vi "Many Stepper Mover Com.vi"() -> (0 "Command text":string[][](array[string]))   [LabVIEW 2019]
uses:
  Stepper Mover.ctl
panel:
  in  "Top or Bottom":T1(radio)
  in  "Initial Value":dbl
  in  "Final Value":dbl
  in  "Number of Interval":dbl
  in  "Generate":bool
  in  "cancel":bool
  in  "next":bool
  in  "Stepper Mover":T2={"extra wait"=0, "Stepper Value"=1.0, "Top or Bottom"=enum."Move to Top Position (deg)"} {"extra wait" min=0; "Stepper Value" format="%#.7e"}
  in  "wait after sweep (sec)":i32
  out "loop array":dbl[][](array[numeric])
  in  "Array":dbl[][](array[numeric]) format="%#_4e"
  # "Stepper Mover (Multiple Input Generator)"
  # "(Stepper Mover.vi needs to be open.)"
  # "generates multiple stepper mover values for the sequence, see belolw.  If you like it click \"Good, use this!\". You can also modify the values directly from the following array."
  # "Value"
  # "Stepper Mover"
  # "(Stepper Mover.vi needs to be open before using this program)"
  # "Value"
  # "seconds"
  # "AND wait extra"
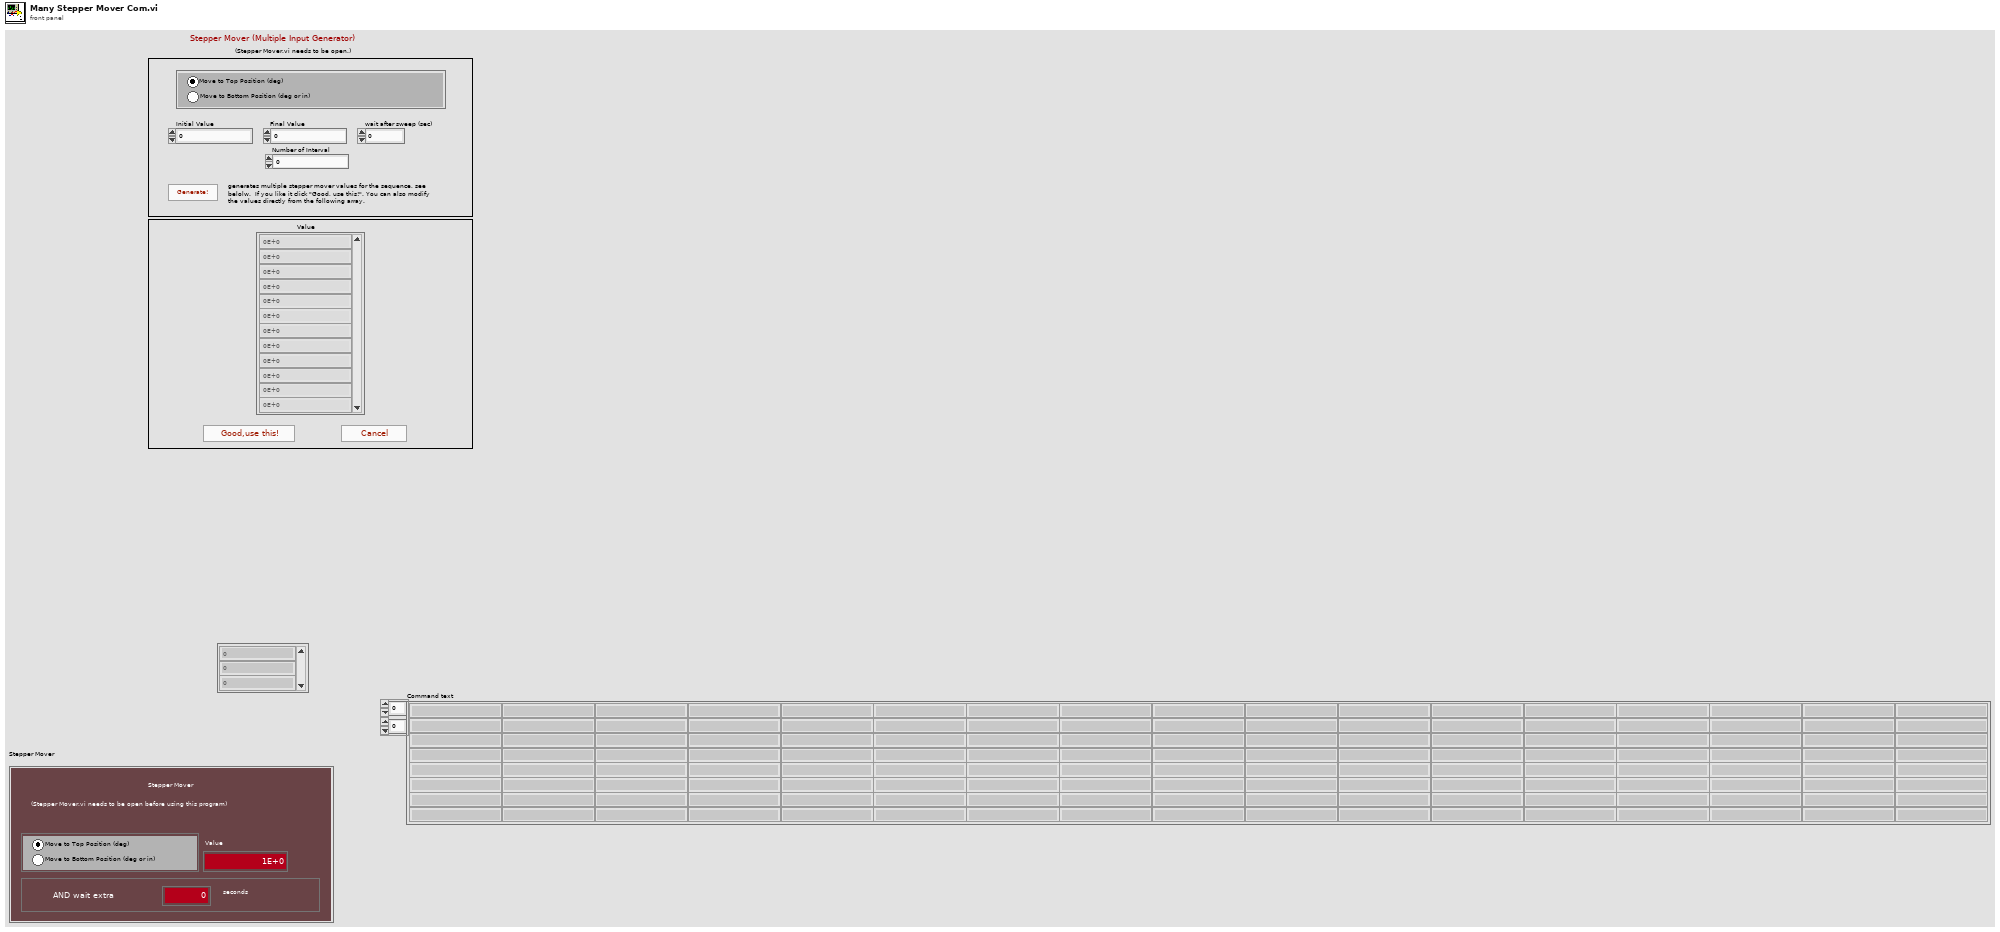
[diagram p1: front panel]
types:
  T1 = enum32{"Move to Top Position (deg)", "Move to Bottom Position (deg or in)"}
  T2 = typedef "Stepper Mover.ctl" = cluster{"extra wait":i32, "Stepper Value":dbl, "Top or Bottom":enum32{"Move to Top Position (deg)", "Move to Bottom Position (deg or in)"}}
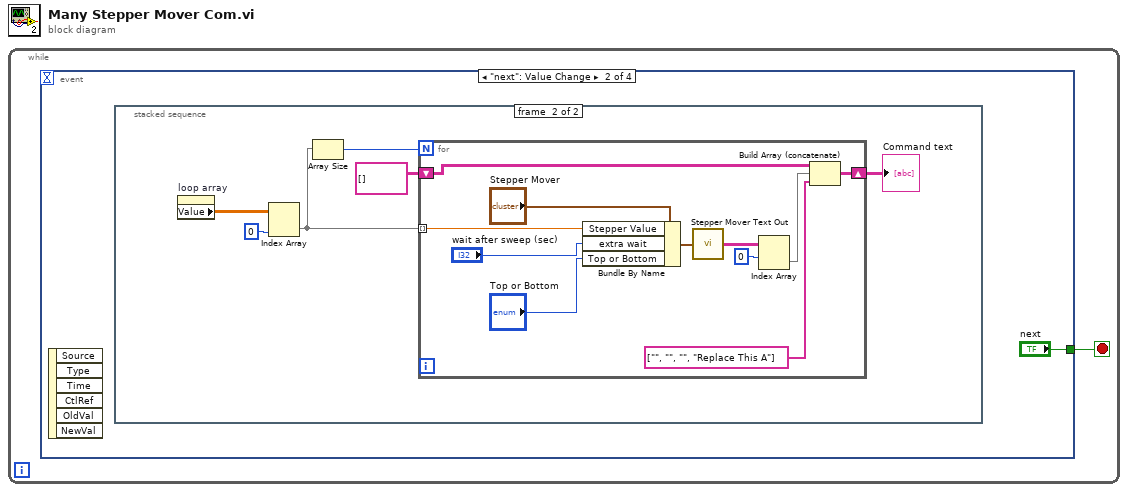
[diagram p0: block diagram]
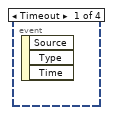
[diagram p2: hidden frame]
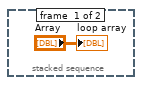
[diagram p3: hidden frame]
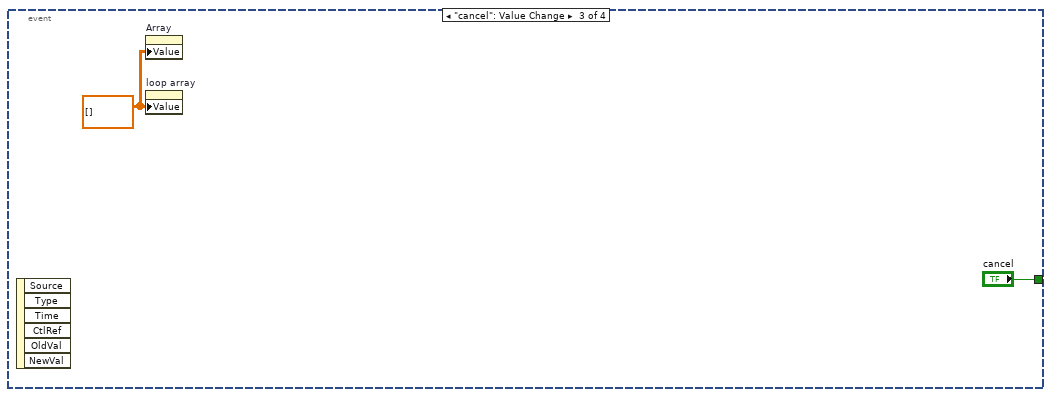
[diagram p4: hidden frame]
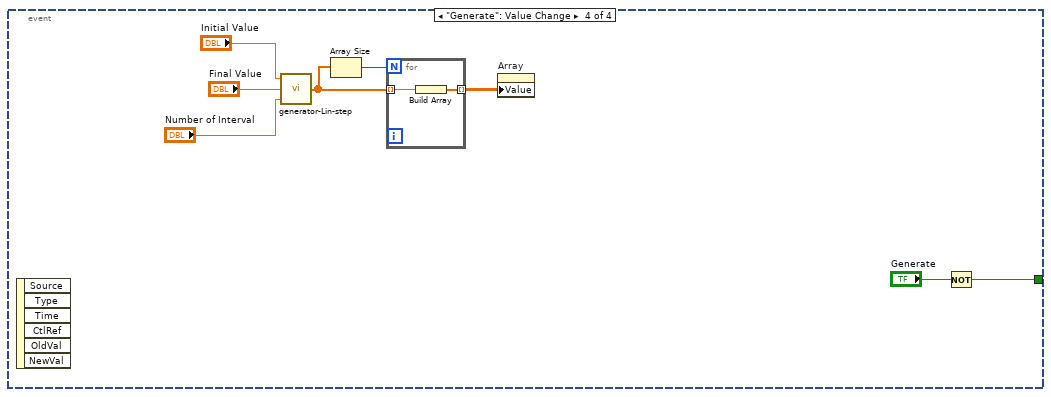
[diagram p5: hidden frame]
diagram:
  n1 = while {
    stop <- w1 stop-if-true
    n2 = event shown="[1] \"next\": Value Change" {
      selector: _ -> [_ _ _ _]
      dyn-events: _ -> [_ _ _ _]
      timeout: _ -> [_ _ _ _]
      tunnel: [_ "next" "cancel" w25] -> w1
      event Timeout {
        n3 = event-data() -> ()  [unwired: 1 in, 3 out]
      }
      event "next": Value Change {
        n4 = event-data() -> ()  [unwired: 1 in, 6 out]
        n5 = stacked-sequence {
          frame #0 {
            "loop array" <- "Array"
          }
          frame #1 {
            n6 = property on="loop array" class="Arr (strict)"() -> ("Value"=w8:dbl[][])  [unwired: 2 in, 2 out]
            n7 = Index Array(array=w8, index (col)=0 ("disabled index (col)")) -> (element=w7:dbl[])  [unwired: 1 in]
            n8 = Array Size(array=w7) -> (size(s)=w6:i32)
            n9 = for {
              N: w6 -> [_]
              tunnel: w7 -> [w11] mode=indexing
              shift-right: [w13] -> w5
              shift-left: string[][] [] -> [w12]
              n10 = Bundle By Name(cluster="Stepper Mover", "Stepper Value"=w11, "extra wait"="wait after sweep (sec)", "Top or Bottom"="Top or Bottom") -> (w19:T2)
              n11 = call "Stepper Mover Text Out.vi"("Stepper Mover"=w19) -> ("Command text"=w17:string[][])
              n12 = Index Array(array=w17, index (row)=0) -> (element=w15:string[])  [unwired: 1 in]
              n13 = Build Array (concatenate)(w12, w15, string[] ["", "", "", "Replace This A"]) -> (w13:string[][])
            }
            "Command text" <- w5
          }
        }
      }
      event "cancel": Value Change {
        w21 = dbl[][] [] ("Array")
        n14 = event-data() -> ()  [unwired: 1 in, 6 out]
        n15 = property on="Array" class="Arr (strict)"("Value"=w21) -> ()  [unwired: 2 in, 2 out]
        n16 = property on="loop array" class="Arr (strict)"("Value"=w21) -> ()  [unwired: 2 in, 2 out]
      }
      event "Generate": Value Change {
        n17 = event-data() -> ()  [unwired: 1 in, 6 out]
        n18 = call "generator-Lin-step.vi"("step"="Number of Interval", "end"="Final Value", "start"="Initial Value") -> ("Array"=w24:dbl[])
        n19 = Array Size(array=w24) -> (size(s)=w26:i32)
        n20 = for {
          N: w26 -> [_]
          tunnel: w24 -> [w32] mode=indexing
          tunnel: [w31] -> w23 mode=indexing
          n21 = Build Array(w32) -> (w31:dbl[])
        }
        n22 = property on="Array" class="Arr (strict)"("Value"=w23) -> ()  [unwired: 2 in, 2 out]
        n23 = Not(x="Generate") -> (.not. x?=w25:bool)
      }
    }
  }
